vi "Set Position Value.vi"(4 "error in (no error)":errorcluster, 5 "new position value":sgl, 6 "Axis In":i16, 7 "Controller Reference":refnum<k7>) -> (0 "error out":errorcluster, 2 "Axis Out":i16, 3 "Controller Reference out":refnum<k7>)   [LabVIEW 2015]
doc: "Resets the current position value for the axis. Default is zero."
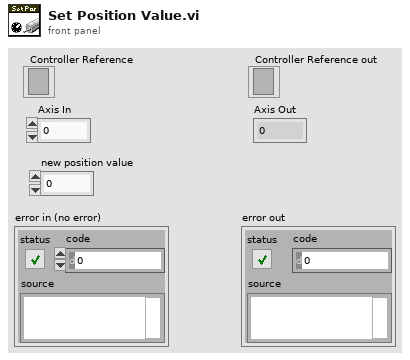
[diagram p1: front panel]
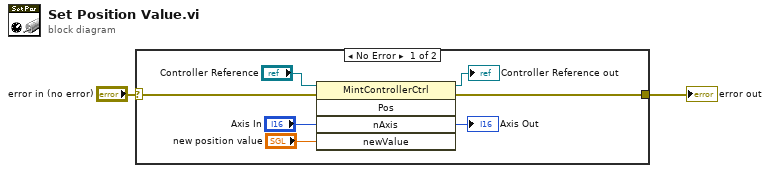
[diagram p0: block diagram]
diagram:
  n1 = case shown="No Error" "error in (no error)" {
    selector: "error in (no error)" -> [w3 w10]
    tunnel: [w7 w10] -> w2
    frame No Error {
      n2 = invoke class="MintControllerCtrl" method="Pos"(reference="Controller Reference", error in=w3, "nAxis"="Axis In", "newValue"="new position value") -> (reference out=→"Controller Reference out":refnum<k7>, error out=w7:errorcluster, "nAxis"=→"Axis Out":i16)  [unwired: 1 in, 2 out]
    }
    frame Error {
    }
  }
  "error out" <- w2
